vi "Clean Build Artifacts.vi"(0 "NI Build Specification in":refnum<class "NI Build Specification_LV.lvclass">, 11 "error in (no error)":errorcluster) -> (4 "NI Build Specification out":refnum<class "NI Build Specification_LV.lvclass">, 15 "error out":errorcluster)   [LabVIEW 2017, in "CL_G3_VIComponentBuilder.lvlib" / "NI Build Specification_LV.lvclass"]
doc: "Removes all built artifacts generated by this export's build. These artifacts are not located in the export directory of the component, but located at the build output specified by the LaBVIEW Project."
uses:
  NI Build Specification_LV.lvclass
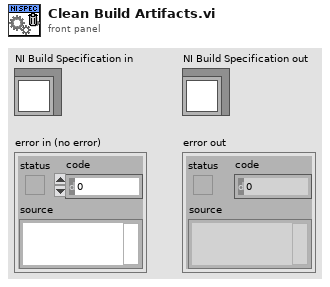
[diagram p1: front panel]
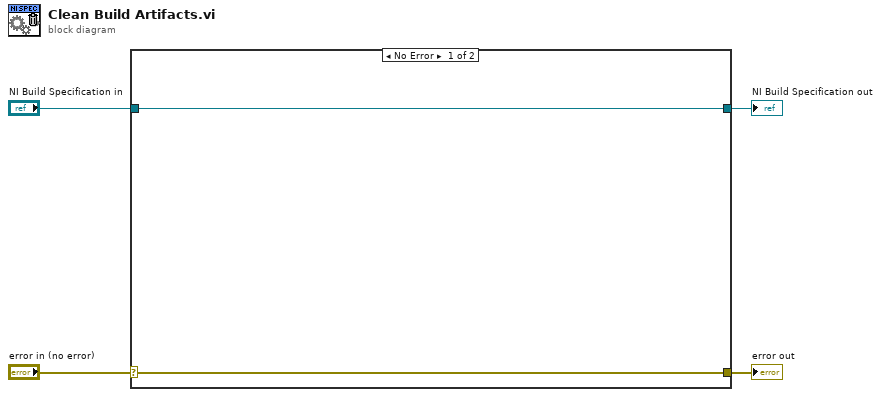
[diagram p0: block diagram]
diagram:
  n1 = case shown="No Error" "error in (no error)" {
    selector: "error in (no error)" -> [w6 w8]
    tunnel: [w6 w8] -> w3
    tunnel: [w5 w7] -> w1
    tunnel: "NI Build Specification in" -> [w5 w7]
    frame No Error {
    }
    frame Error {
    }
  }
  "error out" <- w3
  "NI Build Specification out" <- w1
